vi "JJMCclase9p2.vi"() -> ()   [LabVIEW 2013]
panel:
  out "contador":dbl
  out "numero 50-150":dbl
  # "generar 10 numeros ebtre 50-150 usar un ciclo while para validar que el numero\nse encuentre en ese rango antes de presentarlos\nir contando numeros"
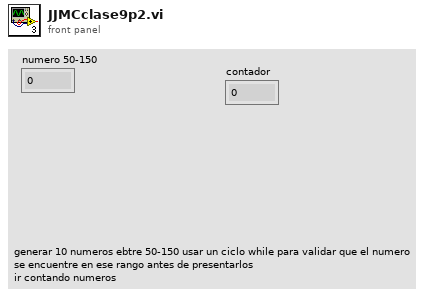
[diagram p1: front panel]
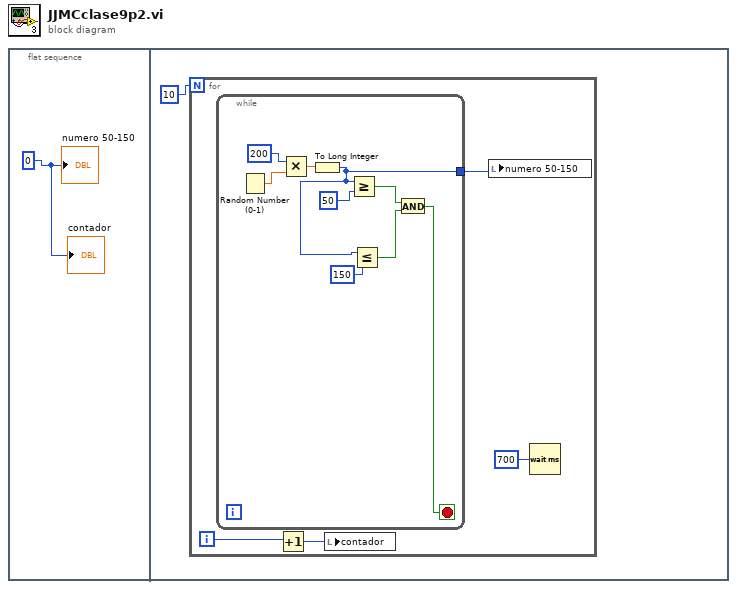
[diagram p0: block diagram]
diagram:
  n1 = flat-sequence {
    frame #0 {
      w1 = 0
      "numero 50-150" <- w1
      "contador" <- w1
    }
    frame #1 {
      n2 = for {
        N: 10 -> [_]
        i -> [w5]
        n3 = while {
          tunnel: [w8] -> w6
          stop <- w7 stop-if-true
          n4 = Random Number (0-1)() -> (number: 0 to 1=w14:dbl)
          n5 = Multiply(x=200, y=w14) -> (x*y=w13:dbl)
          n6 = To Long Integer(number=w13) -> (32bit integer=w8:i32)
          n7 = Greater Or Equal?(x=w8, y=50) -> (x >= y?=w11:bool)
          n8 = Less Or Equal?(x=w8, y=150) -> (x <= y?=w9:bool)
          n9 = And(x=w11, y=w9) -> (x .and. y?=w7:bool)
        }
        n10 = Increment(x=w5) -> (x+1=w4:i32)
        n11 = local write "contador"(w4) -> ()
        n12 = local write "numero 50-150"(w6) -> ()
        n13 = Wait (ms)(milliseconds to wait=700) -> ()  [unwired: 1 out]
      }
    }
  }
